vi "PXI_Host_I8_Read_OldMethod_Benchmark.vi"() -> ()   [LabVIEW 2018]
uses:
  <vilib>/Platform/TimedLoop/XDataNode/timing_clust.ctl
  <vilib>/Platform/TimedLoop/XDataNode/nitl_modes.ctl
  <vilib>/Platform/TimedLoop/XDataNode/wakeup.ctl
  <vilib>/addons/FPGA Advanced Session Resources/LVFPGA Adv Session Resources/OpenByNameSubVI.vi
  <vilib>/rvi/interface/common/dynamic/niFpgaEscapeDelimiterAndNull.vi
  <vilib>/Utility/error.llb/Error Cluster From Error Code.vi
  <vilib>/rvi/errors/niLvFpgaAdjustHostInterfaceError.vi
  <vilib>/FPGAPlugInAG/Dynamic/niLvFpga_Close_Dynamic.vi
  <vilib>/addons/FPGA Advanced Session Resources/LVFPGA Adv Session Resources/OpenByName.xnode
  <vilib>/platform/TimedLoop/XDataNode/XDataNode.xnode
  <vilib>/rvi/interface/nirviReadWriteControl/nirviReadWriteControl.xnode
  <vilib>/rvi/interface/nirviCloseFPGA/nirviCloseFPGA.xnode
  NiFpgaLv.dll
  <vilib>/rvi/interface/Simulation/niFpgaSimulationCallBeginRW.vi
  <vilib>/addons/FPGA Advanced Session Resources/LVFPGA Adv Session Resources/LVFPGAAdvSessionResources.lvlib
  <vilib>/Platform/TimedLoop/XDataNode/XDNodeRunTimeDep.lvlib
panel:
  out "Waveform Graph":dbl[](graph)
  out "Standard Dev":dbl
  out "Arithmetic Mean":dbl
  out "Maximum":dbl
  out "Value out":i8
  out "error out":errorcluster
  # "Recorded time"
  # "3.37551E-5"
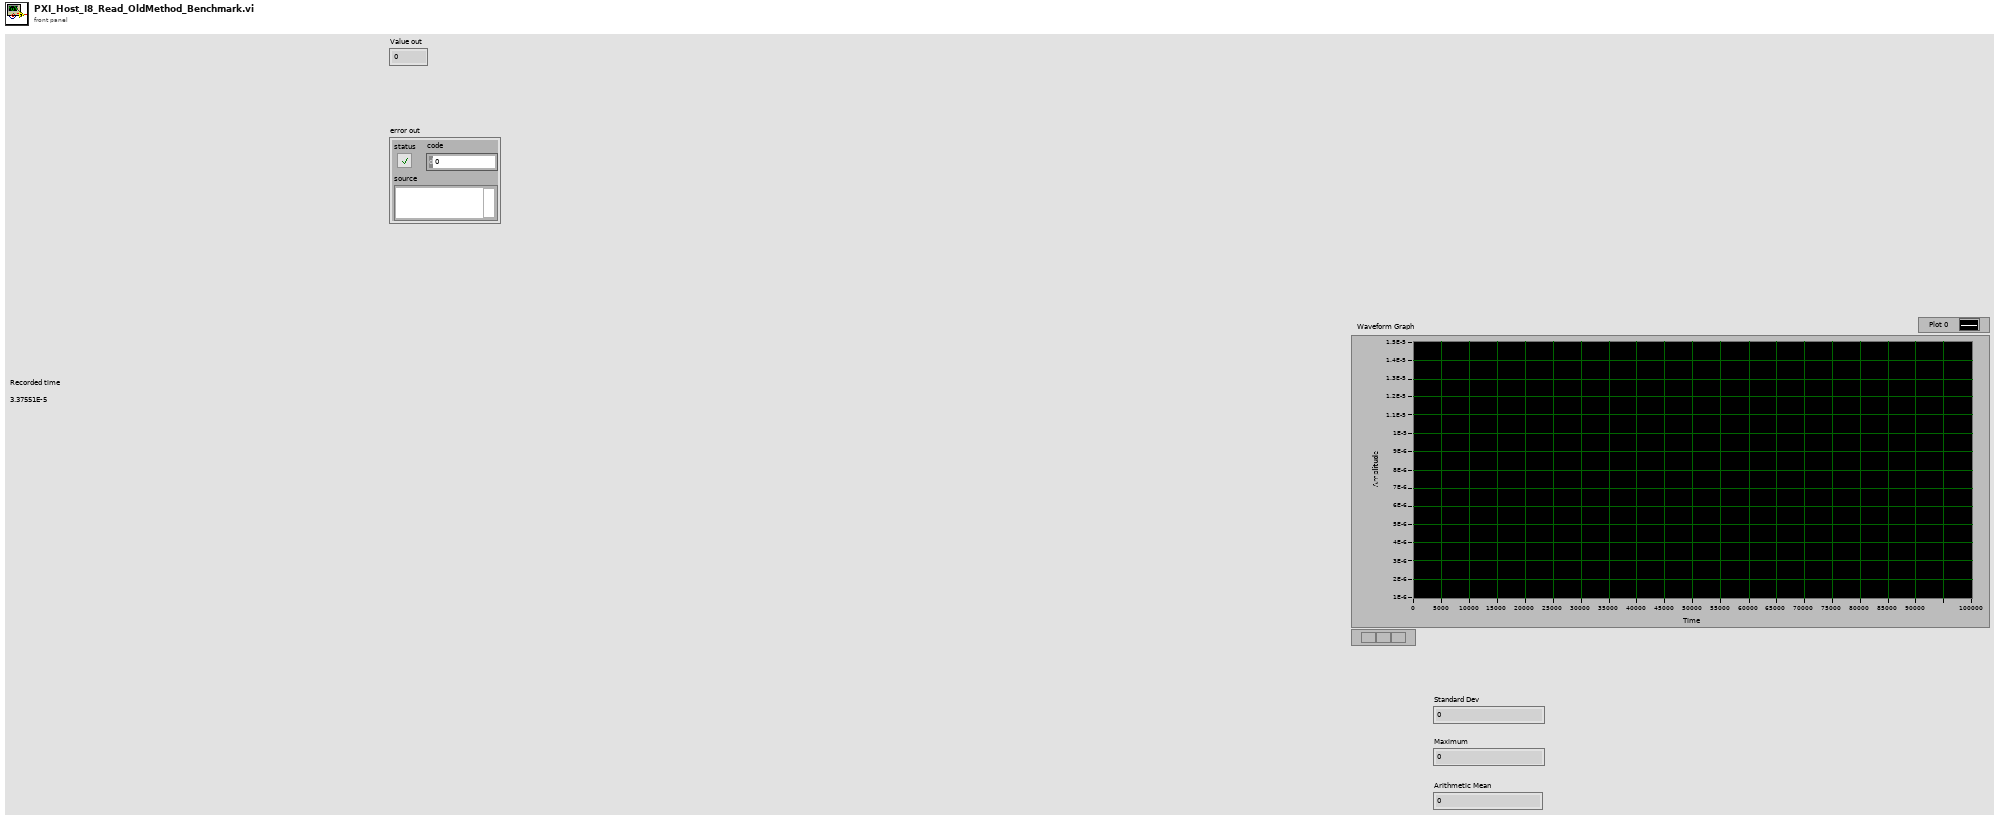
[diagram p1: front panel]
types:
  T1 = typedef "XDNodeRunTimeDep.lvlib/timing_clust.ctl" = cluster{"Expected End [f-1]":u64, "Actual End [f-1]":u64, "Finished Late? [f-1]":bool, "Expected End [i-1]":u64, "Actual End [i-1]":u64, "Finished Late? [i-1]":bool, "Expected Start [i]":u64, "Actual Start [i]":u64, "Expected Start [f]":u64, "Actual Start [f]":u64, "Source Name":string, "Structure Name":string, "Period":i64, "Deadline":i64, "Offset":i64, "Start":i64, "Priority":i32, "Timeout":i32, "Mode":T2, "Wakeup Reason":T3, "Error":errorcluster, "Source Type":string, "Secondary Source Type":string, "Global End Time":u64, "Global Start Time":u64, "Frame Duration":u64, "Iteration Duration":u64, "Assigned CPU":i32, "I/O Scan Engine Mode":u32}
  T2 = typedef "XDNodeRunTimeDep.lvlib/nitl_modes.ctl" = enum32{"No Change", "Process missed periods, maintain original phase", "Discard missed periods, maintain original phase", "Process missed periods, ignore original phase", "Discard missed periods, ignore original phase"}
  T3 = typedef "XDNodeRunTimeDep.lvlib/wakeup.ctl" = enum32{"Normal", "Aborted", "Asynchronous wakeup", "Timing source error", "Timed loop error", "Timeout"}
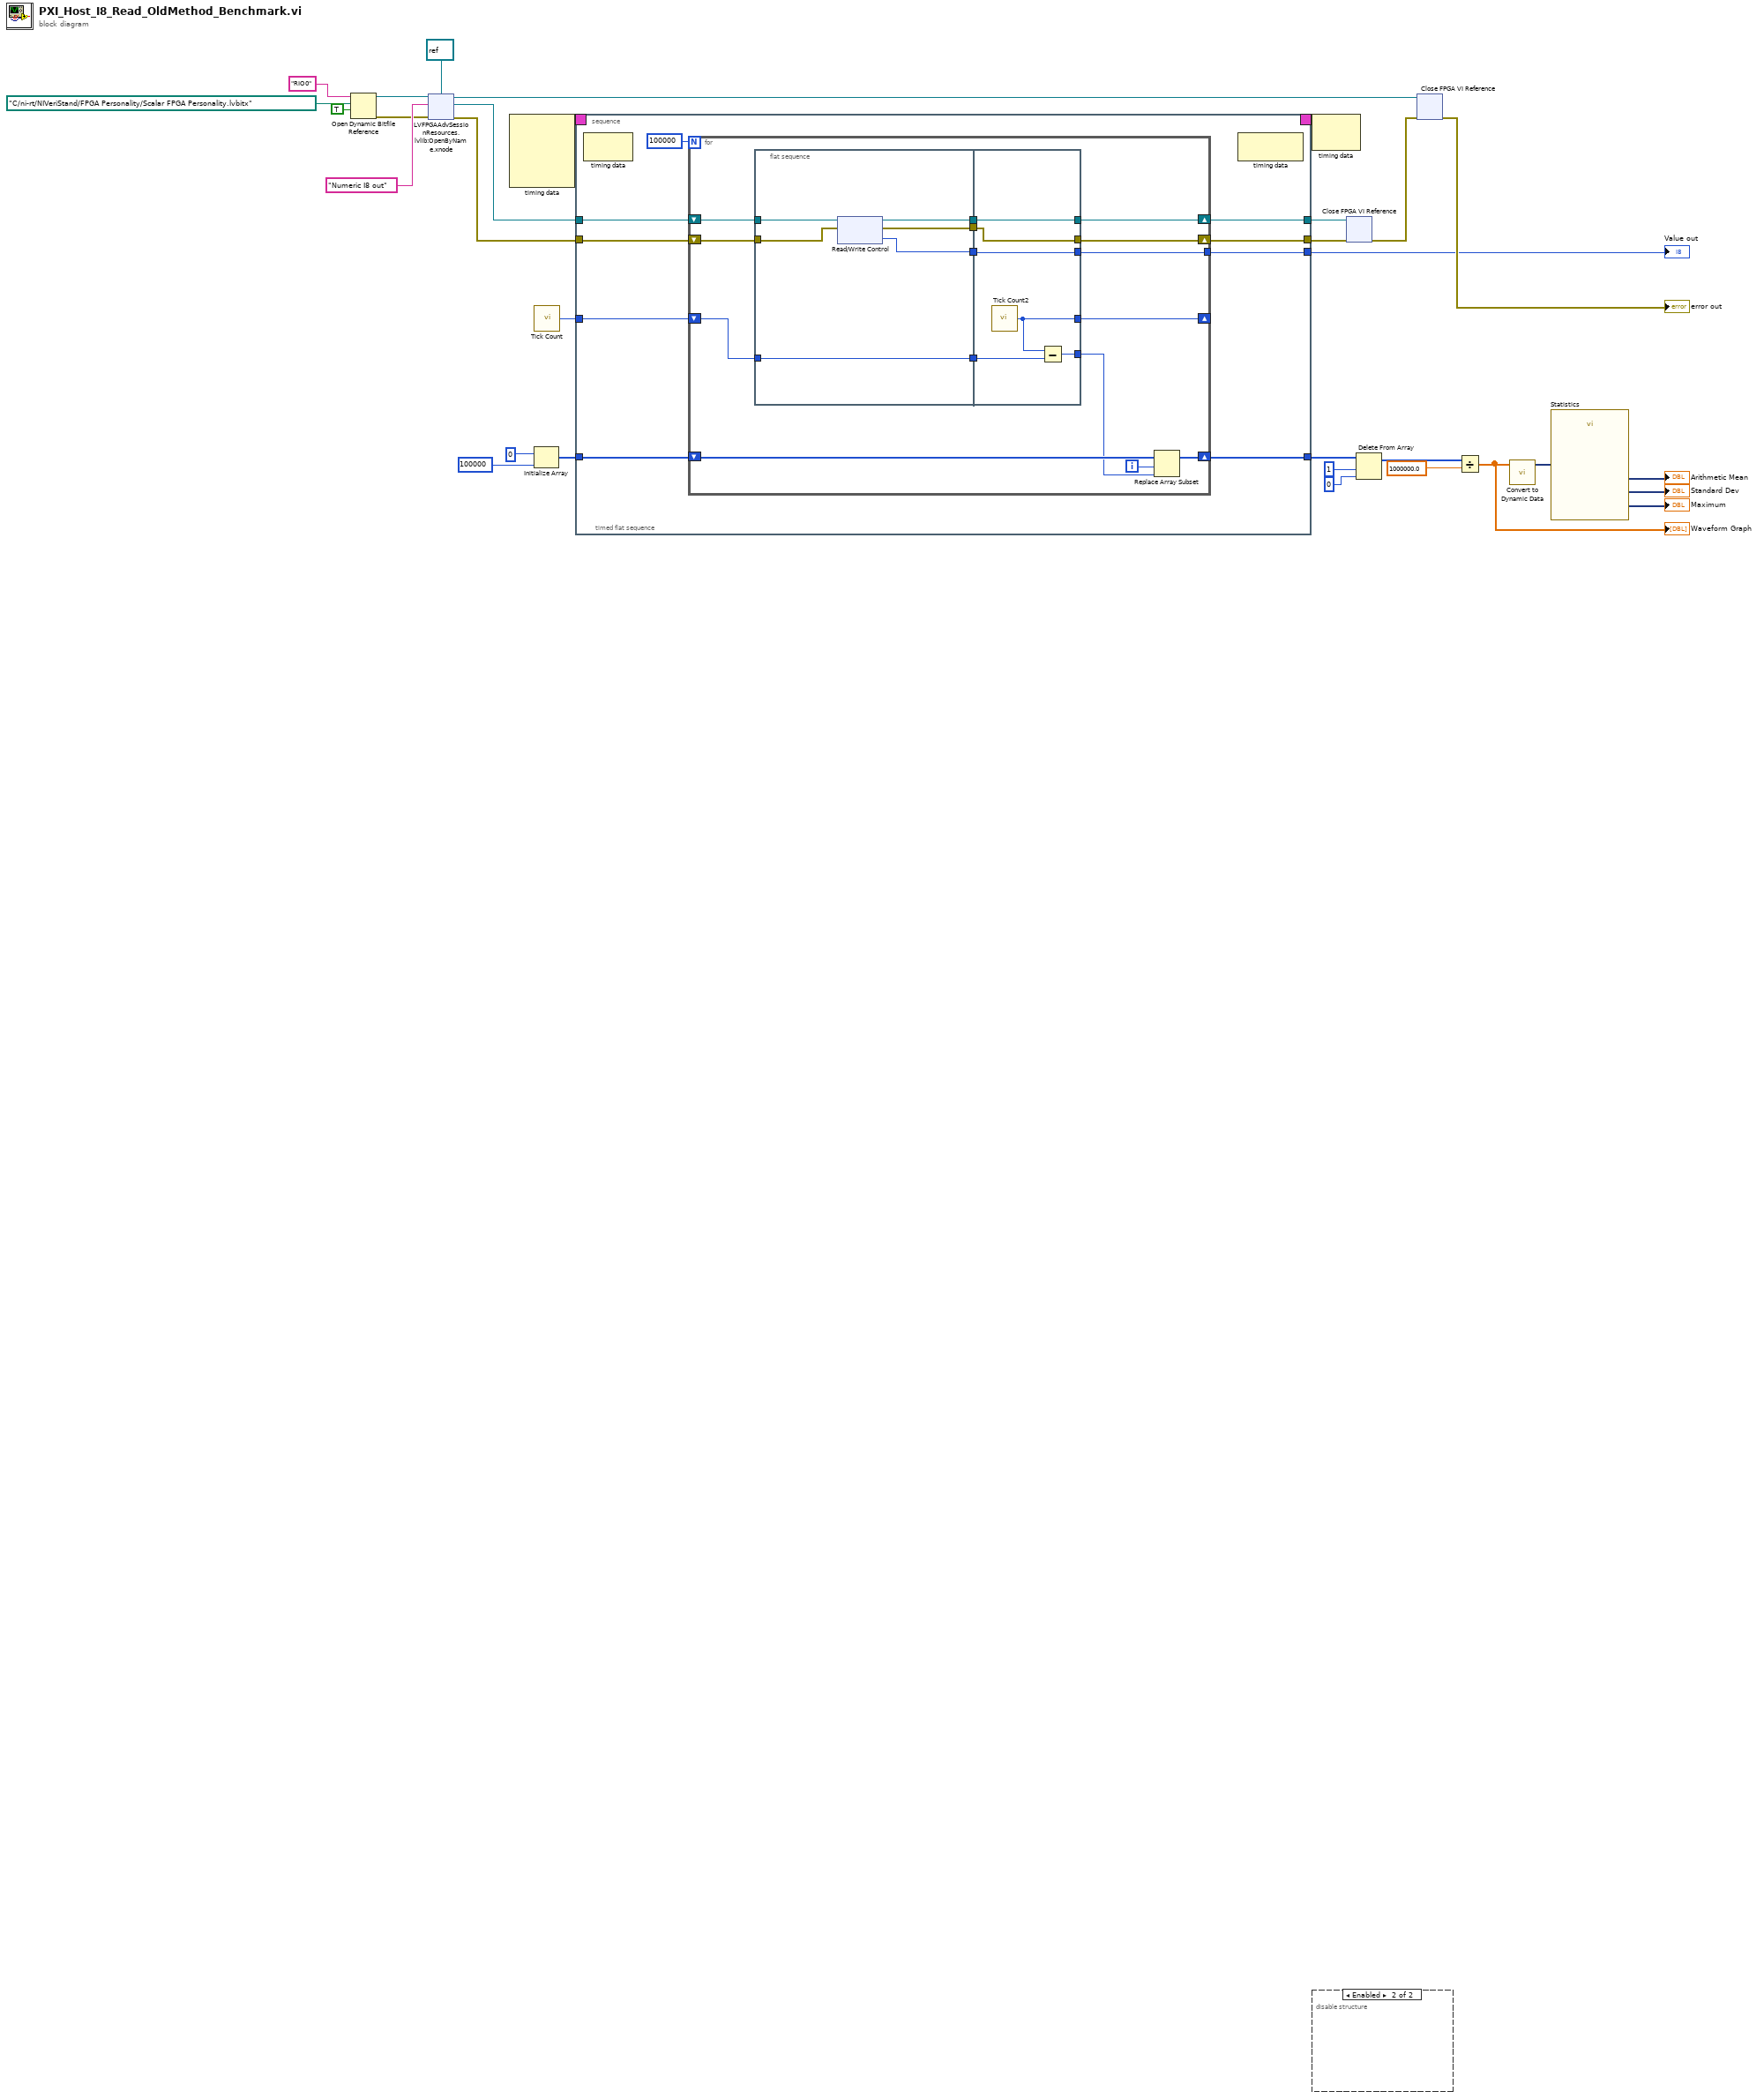
[diagram p0: block diagram]
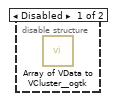
[diagram p2: hidden frame]
diagram:
  n1 = Open Dynamic Bitfile Reference(0:"RIO0" ("Device address"), 1:path "C:/ni-rt/NIVeriStand/FPGA Personality/Scalar FPGA Personality.lvbitx" ("Bitfile path"), 2:TRUE ("Run When Loaded")) -> (5:w28:refnum<k20>, 8:w26:errorcluster)  [unwired: 2 in]
  n2 = xnode "LVFPGAAdvSessionResources.lvlib:OpenByName.xnode"("FPGA VI Reference in"=w28, "Resource name in"="Numeric I8 out", "Single resource reference type in"=refnum<k20> refnum ("Type"), "Error in"=w26) -> ("Single resource reference out"=w24:refnum<k20>, "Error out"=w25:errorcluster, "FPGA VI Reference out"=w21:refnum<k20>)
  n3 = node-c288() -> (w16:T1)  [unwired: 4 in]
  n4 = Initialize Array(u32 0 ("Tick Count(uSec)"), 100000) -> (w11:u32[])
  n5 = call "Tick Count"() -> ("Tick Count(uSec)"=w14:u32)
  n6 = timed-sequence {
    timing: w16 -> [_]
    timing-out: [_] -> w15
    tunnel: w25 -> [w39]
    tunnel: w24 -> [w38]
    tunnel: [w37] -> w19
    tunnel: [w36] -> w18
    tunnel: [w35] -> w17
    tunnel: w14 -> [w34]
    tunnel: w11 -> [w33]
    tunnel: [w32] -> w1
    n7 = timed-flat-sequence {
      tunnel: w39 -> [w48]
      tunnel: w38 -> [w47]
      tunnel: [w46] -> w37
      tunnel: [w45] -> w36
      tunnel: [w44] -> w35
      tunnel: w34 -> [w42]
      tunnel: w33 -> [w41]
      tunnel: [w40] -> w32
      n8 = node-c288() -> ()  [unwired: 1 in, 1 out]
      n9 = for {
        N: 100000 -> [_]
        tunnel: [w56] -> w44
        shift-right: [w58] -> w46
        shift-left: w48 -> [w60]
        shift-right: [w57] -> w45
        shift-left: w47 -> [w59]
        shift-right: [w53] -> _
        shift-left: w42 -> [w55]
        shift-right: [w51] -> w40
        shift-left: w41 -> [w52]
        i -> [w49]
        n10 = flat-sequence {
          tunnel: [w67] -> w63
          tunnel: [w66] -> w62
          tunnel: [w65] -> w61
          tunnel: w59 -> [w69]
          tunnel: w60 -> [w68]
          tunnel: w55 -> [w64]
          tunnel: [w64] -> w54
          tunnel: [w75] -> w50
          tunnel: w63 -> [w74]
          tunnel: [w74] -> w58
          tunnel: w62 -> [w73]
          tunnel: [w73] -> w57
          tunnel: w61 -> [w72]
          tunnel: [w72] -> w56
          tunnel: w54 -> [w71]
          tunnel: [w70] -> w53
          frame #0 {
            n11 = xnode "Read/Write Control"("FPGA VI Reference In"=w69, "error in"=w68) -> ("FPGA VI Reference Out"=w66:refnum<k20>, "error out"=w67:errorcluster, "Value"=w65:i8)
          }
          frame #1 {
            n12 = call "Tick Count2"() -> ("Tick Count(uSec)"=w70:u32)
            n13 = Subtract(x=w70, y=w71) -> (x-y=w75:u32)
          }
        }
        n14 = Replace Array Subset(array=w52, new element=w50, index=w49) -> (w51:u32[])
      }
      n15 = node-c288() -> ()  [unwired: 1 in, 1 out]
    }
  }
  "Value out" <- w17
  n16 = node-c288(w15) -> ()  [unwired: 1 out]
  n17 = disable-structure shown="Enabled" {
    frame Disabled {
      n18 = call <userlib>:"Array of VData to VCluster__ogtk.vi"() -> ()  [unwired: 10 in, 2 out]
    }
    frame Enabled {
    }
  }
  n19 = xnode "Close FPGA VI Reference"("FPGA VI Reference In"=w18, "error in"=w19) -> ("error out"=w22:errorcluster)
  n20 = Delete From Array(array=w1, length=1, index=0) -> (array with subset deleted=w2:u32[])  [unwired: 1 out]
  n21 = xnode "Close FPGA VI Reference"("FPGA VI Reference In"=w21, "error in"=w22) -> ("error out"=→"error out":errorcluster)
  n22 = Divide(x=w2, y=1000000.0) -> (x/y=w3:dbl[])
  "Waveform Graph" <- w3
  n23 = call "Convert to Dynamic Data"("Array"=w3) -> ("Dynamic Data Type"=w10:dynamicdata)  [unwired: 3 in]
  n24 = call "Statistics"("Signals"=w10) -> ("Standard Dev"=→"Standard Dev":dynamicdata, "Arithmetic Mean"=→"Arithmetic Mean":dynamicdata, "Maximum"=→"Maximum":dynamicdata)  [unwired: 23 in, 1 out]
